vi "GetAbort.vi"(8 "error in (no error)":errorcluster, 11 "VI in":refnum<vi>) -> (0 "error out":errorcluster, 2 "Abort":bool, 3 "VI out":refnum<vi>)   [LabVIEW 2017]
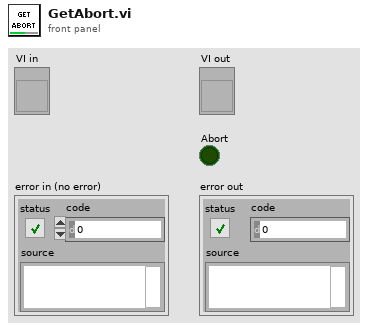
[diagram p1: front panel]
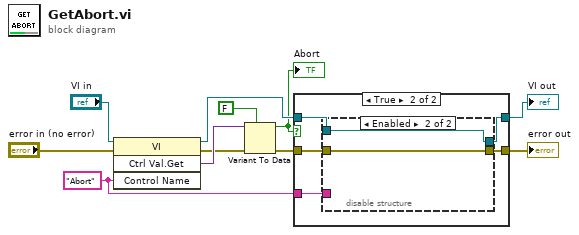
[diagram p0: block diagram]
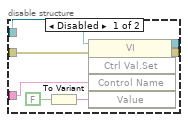
[diagram p3: hidden frame]
diagram:
  w11 = "Abort" ("Control Name")
  n1 = invoke class="VI" method="Ctrl Val.Get"(reference="VI in", error in="error in (no error)", "Control Name"=w11) -> (reference out=w10:refnum<vi>, error out=w7:errorcluster, "Get Control Value Variant"=w9:variant)  [unwired: 1 in, 1 out]
  n2 = Variant To Data(error in=w7, type=FALSE ("Abort"), Variant=w9) -> (data=w5:bool, error out=w6:errorcluster)
  "Abort" <- w5
  n3 = case shown="True" w5 {
    tunnel: w11 -> [_ w18]
    tunnel: w6 -> [w12 w17]
    tunnel: w10 -> [w13 w16]
    tunnel: [w13 w15] -> w2
    tunnel: [w12 w14] -> w1
    frame False {
    }
    frame True {
      n4 = disable-structure shown="Enabled" {
        disable-tunnel: w18 -> [w25 _]
        disable-tunnel: w17 -> [w24 w26]
        disable-tunnel: w16 -> [w23 w27]
        disable-tunnel: [w22 w27] -> w15
        disable-tunnel: [w21 w26] -> w14
        frame Disabled {
          n5 = To Variant(anything=FALSE ("Abort")) -> (Variant=w19:variant)
          n6 = invoke class="VI" method="Ctrl Val.Set"(reference=w23, error in=w24, "Control Name"=w25, "Value"=w19) -> (reference out=w22:refnum<vi>, error out=w21:errorcluster)  [unwired: 1 in, 3 out]
        }
        frame Enabled {
        }
      }
    }
  }
  "error out" <- w1
  "VI out" <- w2
